vi "nCr and nPr using sub VI.vi"() -> ()   [LabVIEW 2024]
panel:
  out "nCr":dbl
  out "nPr":dbl
  in  "r":dbl
  in  "n":dbl
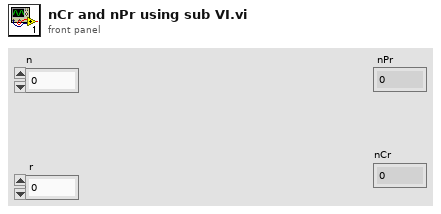
[diagram p1: front panel]
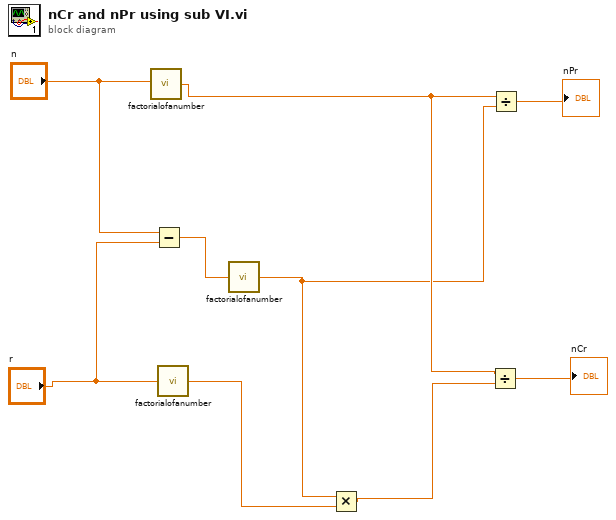
[diagram p0: block diagram]
diagram:
  n1 = call "factorialofanumber.vi"("n"="n") -> ("n!"=w7:dbl)
  n2 = Subtract(x="n", y="r") -> (x-y=w5:dbl)
  n3 = call "factorialofanumber.vi"("n"="r") -> ("n!"=w2:dbl)
  n4 = call "factorialofanumber.vi"("n"=w5) -> ("n!"=w1:dbl)
  n5 = Multiply(x=w1, y=w2) -> (x*y=w3:dbl)
  n6 = Divide(x=w7, y=w3) -> (x/y=→"nCr":dbl)
  n7 = Divide(x=w7, y=w1) -> (x/y=→"nPr":dbl)
